vi "Measurement Parser.vi"(8 "error in (no error)":errorcluster, 9 "Generic Instrument.lvlib:Generic Card.lvclass":refnum<class "Generic Card.lvclass">, 10 "Data Array":dbl[](array[numeric]), 11 "Yokogawa WT500 in":refnum<class "Yokogawa WT500.lvclass">) -> (0 "error out":errorcluster, 2 "Waveform Graph":dynamicdata(graph), 3 "Yokogawa WT500 out":refnum<class "Yokogawa WT500.lvclass">)   [LabVIEW 2014, in "Generic Power Analyzer.lvlib" / "Yokogawa WT500.lvlib" / "Yokogawa WT500.lvclass"]
uses:
  Yokogawa WT500.lvclass
  Generic Instrument/Generic Card/Generic Card.lvclass
  Universal Power Meter/Measured Value Header Control.ctl
  Generic Instrument/Generic Card/Generic Card.lvclass/Generic Card.ctl
  Data Logger/Data Logger.lvclass
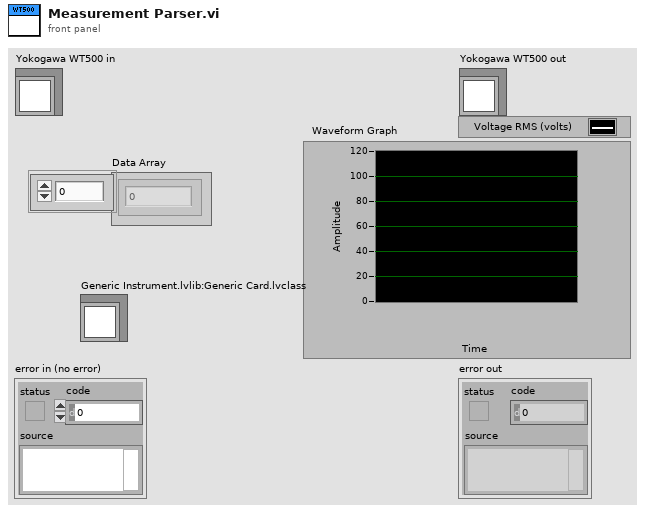
[diagram p1: front panel]
types:
  T1 = typedef "Measured Value Header Control.ctl" = enum16{"Power factor", "Current THD (%)", "Voltage THD (%)", "Amp-Hours", "Energy (Watt-hours)", "Frequency (Herts)", "Power (watts)", "Current RMS (amps)", "Voltage RMS (volts)"}
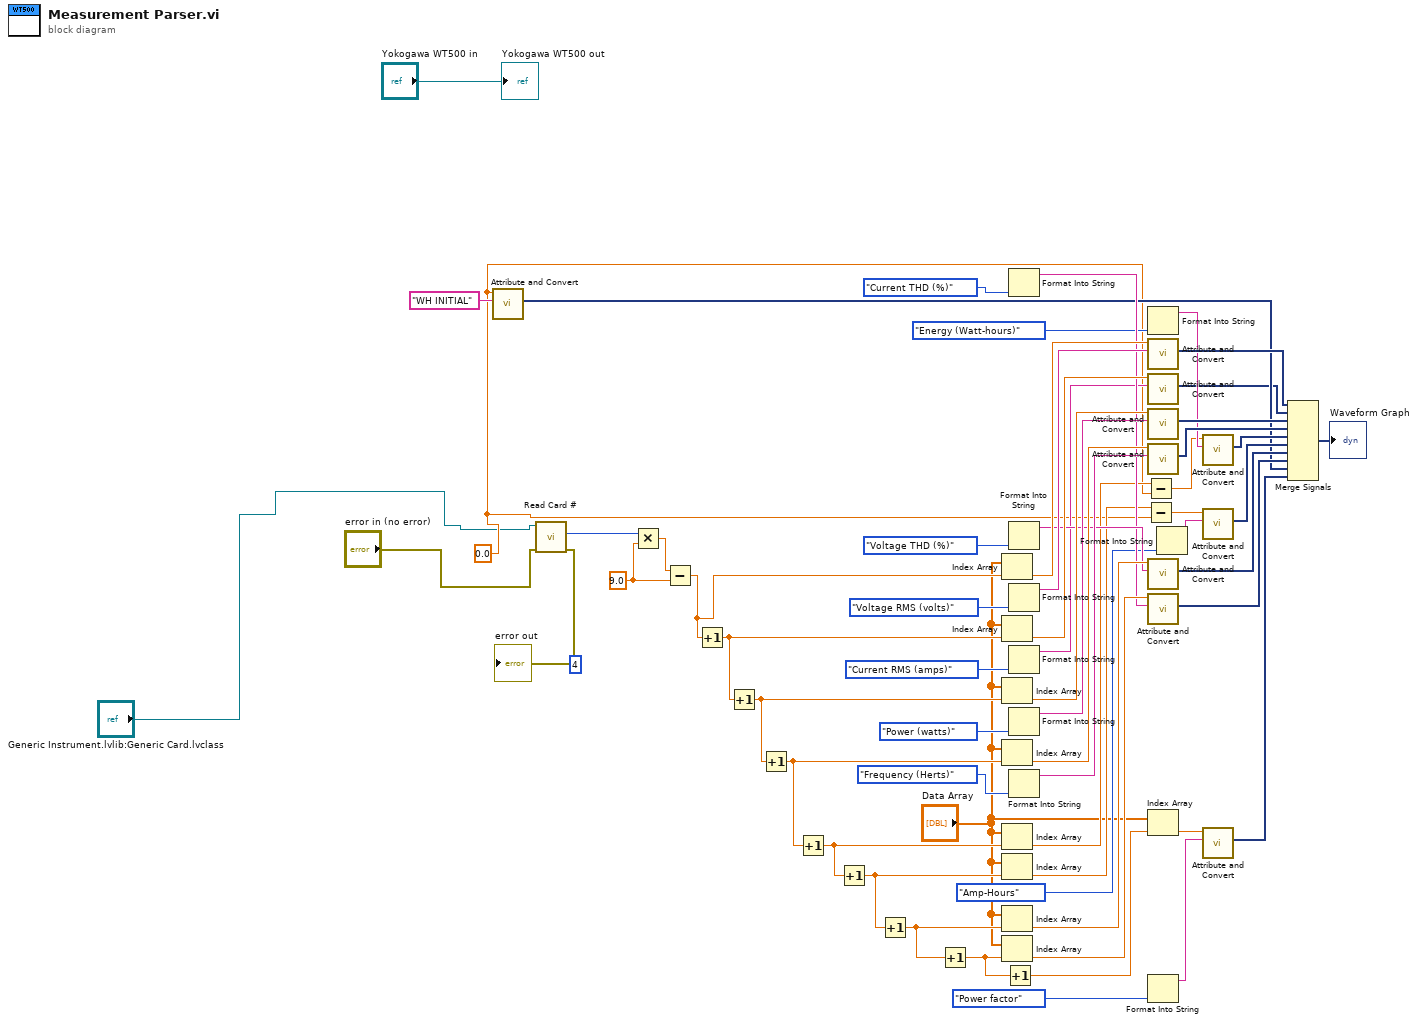
[diagram p0: block diagram]
diagram:
  w3 = 0.0 ("y")
  w6 = 9.0 ("y")
  (unwired) u8 4 ("y")
  n1 = call "Attribute and Convert.vi"("Signal Name"="WH INITIAL", "Number in"=w3) -> ("Dynamic Signal Out"=w23:dynamicdata)  [unwired: 9 in]
  n2 = call "Read Card #.vi"("error in (no error)"="error in (no error)", "Generic Card in"="Generic Instrument.lvlib:Generic Card.lvclass") -> ("error out"=→"error out":errorcluster, "Card #"=w8:u8)  [unwired: 7 in, 1 out]
  n3 = Multiply(x=w8, y=w6) -> (x*y=w7:dbl)
  n4 = Subtract(x=w7, y=w6) -> (x-y=w45:dbl)
  n5 = Increment(x=w45) -> (x+1=w48:dbl)
  n6 = Increment(x=w48) -> (x+1=w50:dbl)
  n7 = Increment(x=w50) -> (x+1=w52:dbl)
  n8 = Increment(x=w52) -> (x+1=w53:dbl)
  n9 = Increment(x=w53) -> (x+1=w40:dbl)
  n10 = Increment(x=w40) -> (x+1=w38:dbl)
  n11 = Increment(x=w38) -> (x+1=w12:dbl)
  n12 = Index Array(array="Data Array", index=w45) -> (element=w46:dbl)
  n13 = Index Array(array="Data Array", index=w48) -> (element=w47:dbl)
  n14 = Index Array(array="Data Array", index=w50) -> (element=w49:dbl)
  n15 = Index Array(array="Data Array", index=w52) -> (element=w51:dbl)
  n16 = Index Array(array="Data Array", index=w53) -> (element=w28:dbl)
  n17 = Index Array(array="Data Array", index=w40) -> (element=w26:dbl)
  n18 = Index Array(array="Data Array", index=w38) -> (element=w44:dbl)
  n19 = Index Array(array="Data Array", index=w12) -> (element=w37:dbl)
  n20 = Increment(x=w12) -> (x+1=w11:dbl)
  n21 = Format Into String(Measured_Value_Header_Control."Current THD (%)" ("Strings")) -> (resulting string=w29:string)  [unwired: 3 in, 1 out]
  n22 = Format Into String(Measured_Value_Header_Control."Voltage THD (%)" ("Strings")) -> (resulting string=w30:string)  [unwired: 3 in, 1 out]
  n23 = Format Into String(Measured_Value_Header_Control."Voltage RMS (volts)" ("Strings")) -> (resulting string=w35:string)  [unwired: 3 in, 1 out]
  n24 = Format Into String(Measured_Value_Header_Control."Current RMS (amps)" ("Strings")) -> (resulting string=w4:string)  [unwired: 3 in, 1 out]
  n25 = Format Into String(Measured_Value_Header_Control."Power (watts)" ("Strings")) -> (resulting string=w34:string)  [unwired: 3 in, 1 out]
  n26 = Format Into String(Measured_Value_Header_Control."Frequency (Herts)" ("Strings")) -> (resulting string=w33:string)  [unwired: 3 in, 1 out]
  n27 = Subtract(x=w28, y=w3) -> (x-y=w27:dbl)
  n28 = Subtract(x=w26, y=w3) -> (x-y=w25:dbl)
  n29 = Format Into String(Measured_Value_Header_Control."Energy (Watt-hours)" ("Strings")) -> (resulting string=w32:string)  [unwired: 3 in, 1 out]
  n30 = call "Attribute and Convert.vi"("Signal Name"=w35, "Number in"=w46) -> ("Dynamic Signal Out"=w54:dynamicdata)  [unwired: 9 in]
  n31 = call "Attribute and Convert.vi"("Signal Name"=w4, "Number in"=w47) -> ("Dynamic Signal Out"=w5:dynamicdata)  [unwired: 9 in]
  n32 = call "Attribute and Convert.vi"("Signal Name"=w34, "Number in"=w49) -> ("Dynamic Signal Out"=w55:dynamicdata)  [unwired: 9 in]
  n33 = call "Attribute and Convert.vi"("Signal Name"=w33, "Number in"=w51) -> ("Dynamic Signal Out"=w56:dynamicdata)  [unwired: 9 in]
  n34 = call "Attribute and Convert.vi"("Signal Name"=w30, "Number in"=w44) -> ("Dynamic Signal Out"=w41:dynamicdata)  [unwired: 9 in]
  n35 = call "Attribute and Convert.vi"("Signal Name"=w29, "Number in"=w37) -> ("Dynamic Signal Out"=w39:dynamicdata)  [unwired: 9 in]
  n36 = Index Array(array="Data Array", index=w11) -> (element=w10:dbl)
  n37 = Format Into String(Measured_Value_Header_Control."Power factor" ("Strings")) -> (resulting string=w14:string)  [unwired: 3 in, 1 out]
  n38 = Format Into String(Measured_Value_Header_Control."Amp-Hours" ("Strings")) -> (resulting string=w31:string)  [unwired: 3 in, 1 out]
  n39 = call "Attribute and Convert.vi"("Signal Name"=w32, "Number in"=w27) -> ("Dynamic Signal Out"=w57:dynamicdata)  [unwired: 9 in]
  n40 = call "Attribute and Convert.vi"("Signal Name"=w31, "Number in"=w25) -> ("Dynamic Signal Out"=w58:dynamicdata)  [unwired: 9 in]
  n41 = call "Attribute and Convert.vi"("Signal Name"=w14, "Number in"=w10) -> ("Dynamic Signal Out"=w9:dynamicdata)  [unwired: 9 in]
  n42 = Merge Signals(w54, w5, w55, w56, w57, w58, w41, w39, w23, w9) -> (→"Waveform Graph":dynamicdata)
  "Yokogawa WT500 out" <- "Yokogawa WT500 in"
